vi "DriveVision.vi"(4 "DriveSmart":bool, 5 "PIDA":T1={"proportional gain (Kc)"=2.0, "integral time (Ti, min)"=0.01, "derivative time (Td, min)"=0.0} {"derivative time (Td, min)" format="%.3f"; "integral time (Ti, min)" format="%.3f"; "proportional gain (Kc)" format="%.3f"}, 6 "TurnSmart":bool=TRUE, 7 "PIDX":T1={"proportional gain (Kc)"=0.04, "integral time (Ti, min)"=0.0, "derivative time (Td, min)"=0.0} {"derivative time (Td, min)" format="%.3f"; "integral time (Ti, min)" format="%.3f"; "proportional gain (Kc)" format="%.3f"}, 8 "MaxErrorA":dbl=1.0, 9 "MaxErrorX":dbl=1.0, 10 "Angle":dbl=0.1 format="%#_13g", 11 "MaxSpeed":dbl=0.3 format="%#_13g") -> (2 "RightOut":dbl, 3 "LeftOut":dbl)   [LabVIEW 2017]
uses:
  Robot Global Data.vi
  <vilib>/addons/control/pid/pid.llb/PID (DBL).vi
  <vilib>/addons/control/pid/NI_PID_pid.lvlib
panel:
  in  "Distance":dbl=2.0 format="%#_13g"
  in  "Speed":dbl format="%#_13g"
  in  "Area":dbl=80.0 format="%#_13g"
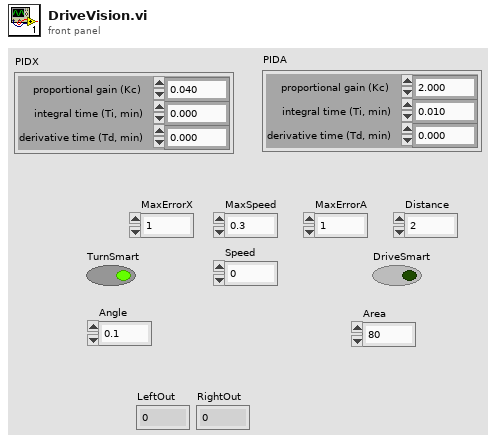
[diagram p1: front panel]
types:
  T1 = cluster{"proportional gain (Kc)":dbl, "integral time (Ti, min)":dbl, "derivative time (Td, min)":dbl}
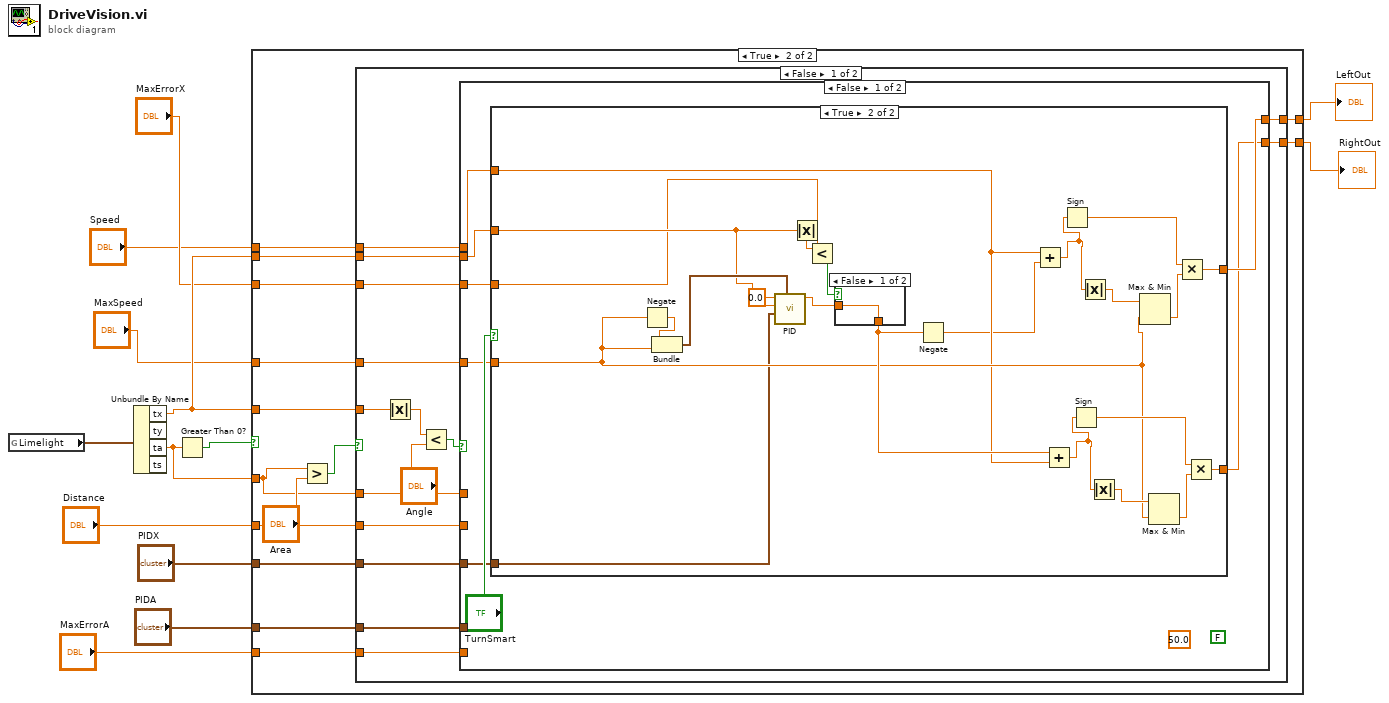
[diagram p0: block diagram]
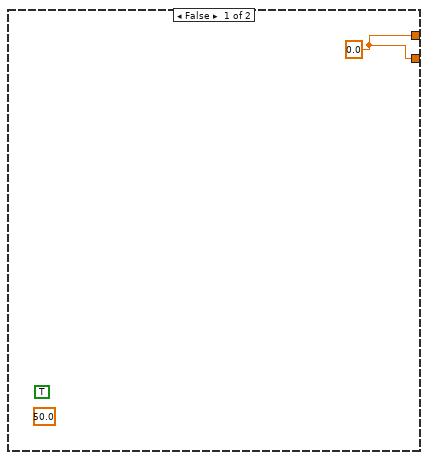
[diagram p2: hidden frame]
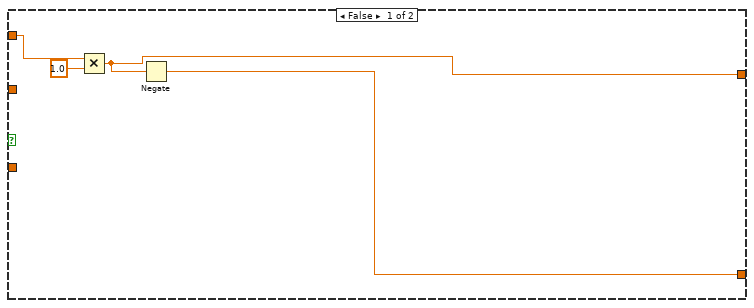
[diagram p3: hidden frame]
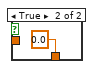
[diagram p4: hidden frame]
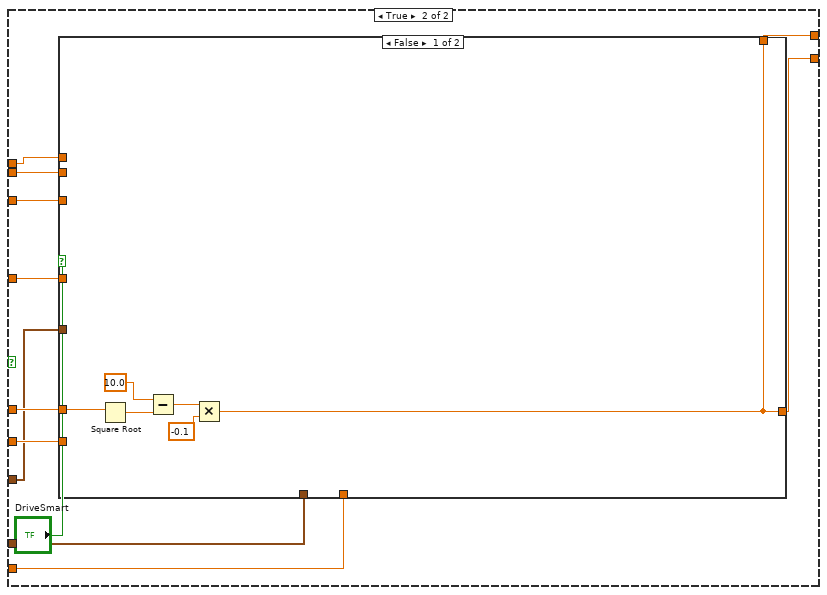
[diagram p5: hidden frame]
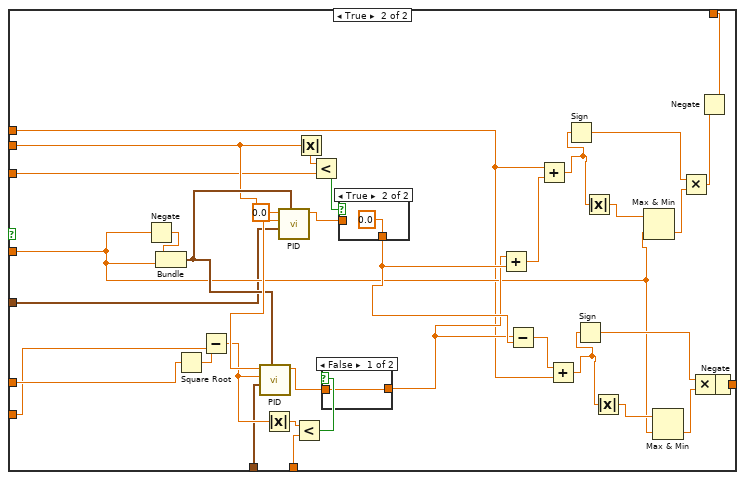
[diagram p6: hidden frame]
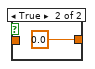
[diagram p7: hidden frame]
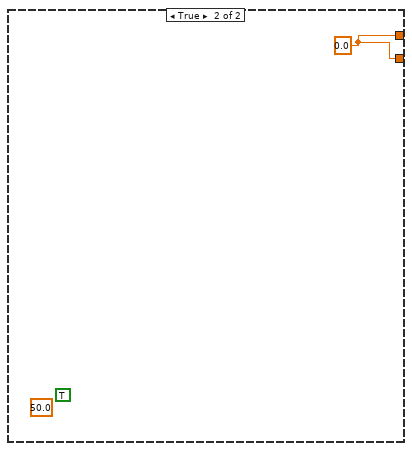
[diagram p9: hidden frame]
diagram:
  n1 = global read "Robot Global Data.vi" "Limelight"() -> (w3:cluster{"tx":dbl, "ty":dbl, "ta":dbl, "ts":dbl})
  n2 = Unbundle By Name(w3) -> ("tx"=w11:dbl, "ta"=w12:dbl)  [unwired: 2 out]
  n3 = Greater Than 0?(x=w12) -> (x > 0?=w13:bool)
  n4 = case shown="True" w13 {
    tunnel: w12 -> [_ w24]
    tunnel: w11 -> [_ w26]
    tunnel: w11 -> [_ w25]
    tunnel: [w14 w23] -> w2
    tunnel: [w14 w22] -> w1
    tunnel: "MaxErrorX" -> [_ w21]
    tunnel: "MaxSpeed" -> [_ w20]
    tunnel: "Speed" -> [_ w19]
    tunnel: "PIDX" -> [_ w18]
    tunnel: "PIDA" -> [_ w17]
    tunnel: "MaxErrorA" -> [_ w16]
    tunnel: "Distance" -> [_ w15]
    frame False {
      w14 = 0.0
      (unwired) 50.0
      (unwired) TRUE
    }
    frame True {
      n5 = Greater?(x=w24, y="Area") -> (0:w27:bool)
      n6 = case shown="False" w27 {
        tunnel: w26 -> [w43 _]
        tunnel: w25 -> [w39 _]
        tunnel: w24 -> [w38 _]
        tunnel: [w37 w139] -> w23
        tunnel: [w36 w139] -> w22
        tunnel: w21 -> [w35 _]
        tunnel: w20 -> [w34 _]
        tunnel: w19 -> [w33 _]
        tunnel: w18 -> [w32 _]
        tunnel: w17 -> [w31 _]
        tunnel: w16 -> [w30 _]
        tunnel: w15 -> [w29 _]
        frame False {
          n7 = Absolute Value(x=w43) -> (abs(x)=w42:dbl)
          n8 = Less?(x=w42, y="Angle") -> (x < y?=w40:bool)
          n9 = case shown="False" w40 {
            tunnel: w39 -> [w48 w92]
            tunnel: w38 -> [_ w91]
            tunnel: [w51 w90] -> w37
            tunnel: [w50 w89] -> w36
            tunnel: w35 -> [w47 w87]
            tunnel: w34 -> [w46 w86]
            tunnel: w33 -> [w45 w81]
            tunnel: w32 -> [w44 w82]
            tunnel: w31 -> [_ w85]
            tunnel: w30 -> [_ w84]
            tunnel: w29 -> [_ w83]
            frame False {
              (unwired) 50.0
              (unwired) FALSE
              n10 = case shown="True" "TurnSmart" {
                tunnel: [w53 w63] -> w51
                tunnel: [w52 w62] -> w50
                tunnel: w48 -> [w55 w61]
                tunnel: w47 -> [_ w60]
                tunnel: w46 -> [_ w59]
                tunnel: w45 -> [_ w58]
                tunnel: w44 -> [_ w57]
                frame False {
                  n11 = Multiply(x=w55, y=1.0) -> (x*y=w53:dbl)
                  n12 = Negate(x=w53) -> (-x=w52:dbl)
                }
                frame True {
                  n13 = Negate(x=w59) -> (-x=w65:dbl)
                  n14 = Bundle(w65, "MaxSpeed"=w59) -> (w64:cluster{dbl, "MaxSpeed":dbl})  [unwired: 1 in]
                  n15 = call-poly <vilib>:"PID.vi"("output range"=w64, "PID gains"=w57, "process variable"=w61, "setpoint"=0.0) -> ("output"=w70:dbl)  [unwired: 6 in, 1 out]
                  n16 = Absolute Value(x=w61) -> (abs(x)=w67:dbl)
                  n17 = Less?(x=w67, y=w60) -> (x < y?=w69:bool)
                  n18 = case shown="False" w69 {
                    tunnel: w70 -> [w79 _]
                    tunnel: [w79 0.0] -> w68
                    frame False {
                    }
                    frame True {
                    }
                  }
                  n19 = Negate(x=w68) -> (-x=w56:dbl)
                  n20 = Add(x=w58, y=w56) -> (x+y=w75:dbl)
                  n21 = Add(x=w68, y=w58) -> (x+y=w71:dbl)
                  n22 = Sign(1:w75) -> (0:w76:dbl)
                  n23 = Sign(1:w71) -> (0:w72:dbl)
                  n24 = Absolute Value(x=w75) -> (abs(x)=w78:dbl)
                  n25 = Absolute Value(x=w71) -> (abs(x)=w74:dbl)
                  n26 = Max & Min(x=w78, y=w59) -> (min(x,y)=w77:dbl)  [unwired: 1 out]
                  n27 = Max & Min(x=w74, y=w59) -> (min(x,y)=w73:dbl)  [unwired: 1 out]
                  n28 = Multiply(x=w76, y=w77) -> (x*y=w63:dbl)
                  n29 = Multiply(x=w72, y=w73) -> (x*y=w62:dbl)
                }
              }
            }
            frame True {
              n30 = case shown="False" "DriveSmart" {
                tunnel: w92 -> [_ w111]
                tunnel: w91 -> [w98 w110]
                tunnel: [w93 w100] -> w90
                tunnel: [w93 w99] -> w89
                tunnel: w87 -> [_ w107]
                tunnel: w86 -> [_ w106]
                tunnel: w85 -> [_ w105]
                tunnel: w84 -> [_ w104]
                tunnel: w83 -> [_ w103]
                tunnel: w82 -> [_ w102]
                tunnel: w81 -> [_ w101]
                frame False {
                  n31 = Square Root(x=w98) -> (sqrt(x)=w96:dbl)
                  n32 = Subtract(x=10.0, y=w96) -> (x-y=w95:dbl)
                  n33 = Multiply(x=w95, y=-0.1) -> (x*y=w93:dbl)
                }
                frame True {
                  w119 = 0.0 ("setpoint")
                  n34 = Negate(x=w106) -> (-x=w113:dbl)
                  n35 = Bundle(w113, "MaxSpeed"=w106) -> (w112:cluster{dbl, "MaxSpeed":dbl})  [unwired: 1 in]
                  n36 = Square Root(x=w110) -> (sqrt(x)=w120:dbl)
                  n37 = Subtract(x=w120, y=w103) -> (x-y=w117:dbl)
                  n38 = call-poly <vilib>:"PID.vi"("output range"=w112, "PID gains"=w105, "process variable"=w117, "setpoint"=w119) -> ("output"=w118:dbl)  [unwired: 6 in, 1 out]
                  n39 = Absolute Value(x=w117) -> (abs(x)=w116:dbl)
                  n40 = call-poly <vilib>:"PID.vi"("output range"=w112, "PID gains"=w102, "process variable"=w111, "setpoint"=w119) -> ("output"=w124:dbl)  [unwired: 6 in, 1 out]
                  n41 = Less?(x=w116, y=w104) -> (x < y?=w115:bool)
                  n42 = Absolute Value(x=w111) -> (abs(x)=w121:dbl)
                  n43 = Less?(x=w121, y=w107) -> (x < y?=w123:bool)
                  n44 = case shown="False" w115 {
                    tunnel: w118 -> [w135 _]
                    tunnel: [w135 0.0] -> w114
                    frame False {
                    }
                    frame True {
                    }
                  }
                  n45 = case shown="True" w123 {
                    tunnel: w124 -> [w137 _]
                    tunnel: [w137 0.0] -> w122
                    frame False {
                    }
                    frame True {
                    }
                  }
                  n46 = Add(x=w114, y=w122) -> (x+y=w134:dbl)
                  n47 = Subtract(x=w114, y=w122) -> (x-y=w125:dbl)
                  n48 = Add(x=w101, y=w134) -> (x+y=w130:dbl)
                  n49 = Add(x=w125, y=w101) -> (x+y=w126:dbl)
                  n50 = Sign(1:w130) -> (0:w131:dbl)
                  n51 = Sign(1:w126) -> (0:w127:dbl)
                  n52 = Absolute Value(x=w130) -> (abs(x)=w133:dbl)
                  n53 = Absolute Value(x=w126) -> (abs(x)=w129:dbl)
                  n54 = Max & Min(x=w133, y=w106) -> (min(x,y)=w132:dbl)  [unwired: 1 out]
                  n55 = Max & Min(x=w129, y=w106) -> (min(x,y)=w128:dbl)  [unwired: 1 out]
                  n56 = Multiply(x=w131, y=w132) -> (x*y=w109:dbl)
                  n57 = Multiply(x=w127, y=w128) -> (x*y=w108:dbl)
                  n58 = Negate(x=w109) -> (-x=w100:dbl)
                  n59 = Negate(x=w108) -> (-x=w99:dbl)
                }
              }
            }
          }
        }
        frame True {
          w139 = 0.0
          (unwired) 50.0
          (unwired) TRUE
        }
      }
    }
  }
  "LeftOut" <- w2
  "RightOut" <- w1
